vi "Begin.vi"(8 "error in":errorcluster) -> (0 "error out":errorcluster)   [LabVIEW 2014]
doc: "Called before other user functions, this VI is expected to open initial I/O refnums, load in file data, and do all program initialization. Notice that the <B>error out</B> terminal is simply used for data flow. Wiring it to other structures or subVIs ensures that this VI runs first."
uses:
  <vilib>/Rock Robotics/WPI/DriverStation/WPI_DriverStationRobotMode2.ctl
  Robot Global Data.vi
  <vilib>/Rock Robotics/Network Tables/SD Write String Array.vi
panel:
  out "filenames":string[](array[string])
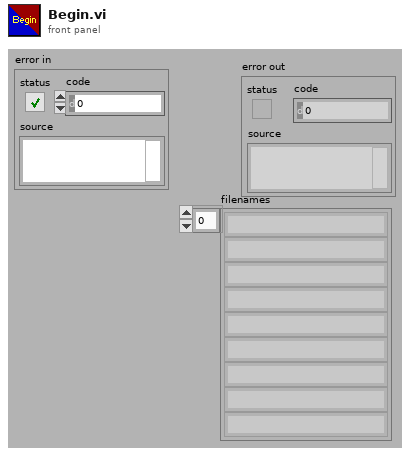
[diagram p1: front panel]
types:
  T1 = typedef "WPI_DriverStationRobotMode2.ctl" = enum16{"Autonomous Disabled", "Autonomous Enabled", "Teleop Disabled", "Teleop Enabled", "Disconnected", "Finish", "Test Disabled", "Test Enabled", "Emergency Stopped"}
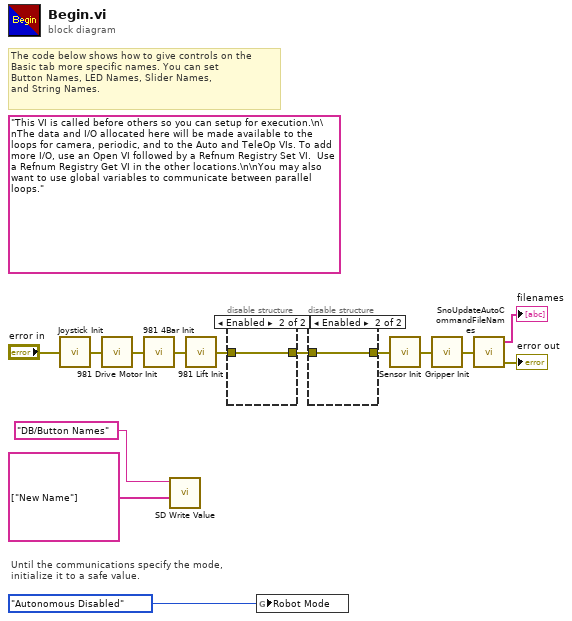
[diagram p0: block diagram]
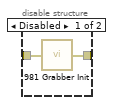
[diagram p2: hidden frame]
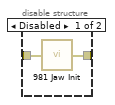
[diagram p3: hidden frame]
diagram:
  (unwired) "This VI is called before others so you can setup for execution.\n\nThe data and I/O allocated here will be made available to the loops for camera, periodic, and to the Auto and TeleOp VIs. To add more I/O, use an Open VI followed by a Refnum Registry Set VI.  Use a Refnum Registry Get VI in the other locations.\n\nYou may also want to use global variables to communicate between parallel loops."
  # "The code below shows how to give controls on the\nBasic tab more specific names. You can set\nButton Names, LED Names, Slider Names,\nand String Names."
  # "Until the communications specify the mode,\ninitialize it to a safe value."
  n1 = call "Joystick Init.vi"("error in"="error in") -> ("error out"=w11:errorcluster)
  n2 = call "981 Drive Motor Init.vi"("error in"=w11) -> ("error out"=w9:errorcluster)
  n3 = call "981 4Bar Init.vi"("error in"=w9) -> ("error out"=w8:errorcluster)
  n4 = call-poly <vilib>:"SD Write Value.vi"("String Array"=string[] ["New Name"], "Name"="DB/Button Names") -> ()  [unwired: 8 in, 2 out]
  n5 = call "981 Lift Init.vi"("error in"=w8) -> ("error out"=w7:errorcluster)
  n6 = disable-structure shown="Enabled" {
    disable-tunnel: w7 -> [w16 w17]
    disable-tunnel: [w15 w17] -> w6
    frame Disabled {
      n7 = call "981 Grabber Init.vi"("error in"=w16) -> ("error out"=w15:errorcluster)
    }
    frame Enabled {
    }
  }
  n8 = global write "Robot Global Data.vi" "Robot Mode"(WPI_DriverStationRobotMode2."Autonomous Disabled" ("Robot Mode")) -> ()
  n9 = disable-structure shown="Enabled" {
    disable-tunnel: w6 -> [w19 w20]
    disable-tunnel: [w18 w20] -> w5
    frame Disabled {
      n10 = call "981 Jaw Init.vi"("error in"=w19) -> ("error out"=w18:errorcluster)
    }
    frame Enabled {
    }
  }
  n11 = call "Sensor Init.vi"("error in"=w5) -> ("error out"=w2:errorcluster)
  n12 = call "Gripper Init.vi"("error in (no error)"=w2) -> ("error out"=w1:errorcluster)
  n13 = call "SnoUpdateAutoCommandFileNames.vi"("error in (no error)"=w1) -> ("error out"=→"error out":errorcluster, "filenames"=→"filenames":string[])
